vi "RSZVB Overwrite Noise Figure Channel Settings.vi"(8 "error in (no error)":errorcluster {"code" format="%.0x"}, 9 "Trace Name (\"Trc1\")":string="Trc1", 10 "Channel (1)":i32=1, 11 "VISA session":refnum<visa-resource-name>) -> (0 "error out":errorcluster {"code" format="%.0x"}, 3 "dup VISA session":refnum<visa-resource-name>)   [LabVIEW 2011]
doc: "This VI overwrites the current channel settings with the ones that were used during the active (previously performed) noise figure calibration. The referenced trace must show the noise figure of a device.\n\nNote(s):\n\n(1) This VI is available only with option R&S ZVAB-K30.\n\nRemote-control command(s):\nCALCulate<Ch>:PARameter:NFIGure:CSETtings"
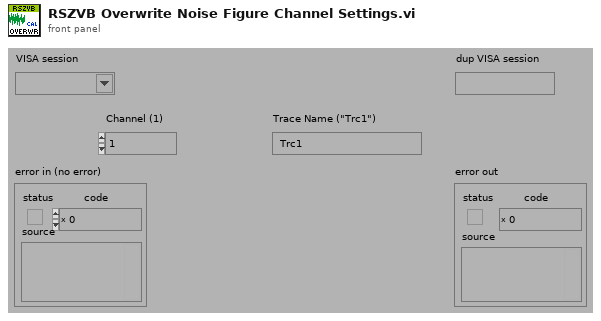
[diagram p1: front panel]
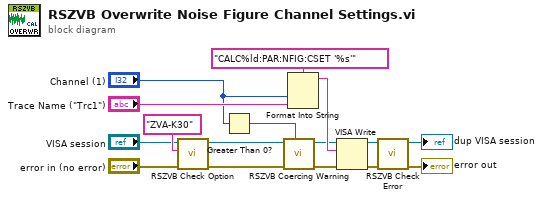
[diagram p0: block diagram]
diagram:
  n1 = call "RSZVB Check Option.vi"("error in (no error)"="error in (no error)", "Options"="ZVA-K30", "VISA session"="VISA session") -> ("error out"=w7:errorcluster, "dup VISA session"=w8:refnum<visa-resource-name>)  [unwired: 7 in]
  n2 = Greater Than 0?(x="Channel (1)") -> (x > 0?=w16:bool)
  n3 = call "RSZVB Coercing Warning.vi"("In Range?"=w16, "error in (no error)"=w7, "VISA session"=w8) -> ("error out"=w12:errorcluster, "dup VISA session"=w11:refnum<visa-resource-name>)  [unwired: 7 in]
  n4 = Format Into String(format string="CALC%ld:PAR:NFIG:CSET '%s'", "Channel (1)", "Trace Name (\"Trc1\")") -> (resulting string=w13:string)  [unwired: 2 in, 1 out]
  n5 = VISA Write(VISA resource name=w11, write buffer=w13, error in (no error)=w12) -> (VISA resource name out=w14:refnum<visa-resource-name>, error out=w15:errorcluster)  [unwired: 1 out]
  n6 = call "RSZVB Check Error.vi"("error in (no error)"=w15, "VISA session"=w14) -> ("error out"=→"error out":errorcluster, "dup VISA session"=→"dup VISA session":refnum<visa-resource-name>)  [unwired: 8 in]
